vi "Bertta_v09_95.vi"() -> ()   [LabVIEW 2015]
panel:
  out "element":bool
  out "Started:":string
  in  "SHUTDOWN":bool
  in  "MASTER CONTROL":bool
  in  "Tab Control":T1(tab)
  out "Output File":path caption="selected path"
  in  "Browse folder":path=path "" caption="start path"
  in  "Read Seq":bool
  in  "Save Seq":bool
  in  "Configuration file":path=path "C:/Users/shresplab/Desktop/BerttaConfiguration.lvm" caption="Filename"
  in  "OK Button 2":bool
  out "Boolean":bool
  in  "User (initials)":string
  in  "Project name":string
  in  "Description":string
  out "PUMP1":bool
  out "Target amount":dbl
  out "Scale weight":dbl
  out "Amount now":dbl
  out "Flow rate":dbl
  out "Time to target":dbl format="%<%H:%M:%S>t"
  out "Current step":dbl
  out "Target":dbl
  out "Amount now":dbl
  out "Amount now":dbl
  out "Target":dbl
  out "Current step":dbl
  out "Time to target":dbl format="%<%H:%M:%S>t"
  out "Flow rate":dbl
  out "Amount now":dbl
  out "Scale weight":dbl
  out "Target amount":dbl
  out "PUMP2":bool
  out "Sensor OK 6":bool
  out "Sensor OK 5":bool
  out "Sensor OK 4":bool
  out "Sensor OK 3":bool
  in  "OK Button":bool
  in  "Add comment":string
  out "PUMP3":bool
  out "Target amount":dbl
  out "Scale weight":dbl
  out "Amount now":dbl
  out "Flow rate":dbl
  out "Time to target":dbl format="%<%H:%M:%S>t"
  out "Current step":dbl
  out "Target":dbl
  out "Amount now":dbl
  out "Tr":dbl
  out "Tj in":dbl
  out "Tj out":dbl
  out "T set":dbl
  out "Current step":i32
  out "RPM":dbl
  out "Torque 2":dbl
  out "Waveform Chart 5":dynamicdata(graph)
  out "Waveform Chart 6":dynamicdata(graph)
  out "Waveform Chart 7":dynamicdata(graph)
  in  "Tab Control 2":T2(tab)
  out "Waveform Chart 3":dynamicdata(graph)
  out "Waveform Chart 8":dynamicdata(graph)
  out "Waveform Chart 11":dynamicdata(graph)
  out "Waveform Chart 13":dynamicdata(graph)
  out "Waveform Chart 9":dynamicdata(graph)
  out "Table":string[][](table)=[["14.8.2017 18.06.59", "0,000000", "417,670000", "-0,150000", "1,000000", "22,220000", "23,366837", "23,574959", "23,985852", "23,690000", "240,000000", "4,000000", "0,000000", "397,000000", "-397,000000", "1,000000"], ["14.8.2017 18.07.06", "0,000000", "417,640000", "-0,120000", "1,000000", "22,220000", "23,763115", "23,906257", "23,985694", "23,680000", "240,000000", "4,000000", "0,000000", "397,000000", "-397,000000", "1,000000"], ["14.8.2017 18.07.13", "0,000000", "417,640000", "-0,120000", "1,000000", "22,220000", "23,965922", "24,013440", "23,984906", "23,670000", "240,000000", "4,100000", "3,000000", "397,000000", "-397,000000", "1,000000"], ["14.8.2017 18.07.21", "0,000000", "417,640000", "-0,120000", "1,000000", "22,220000", "23,943860", "23,900110", "23,987113", "23,670000", "240,000000", "4,000000", "0,000000", "397,000000", "-397,000000", "1,000000"], ["14.8.2017 18.07.28", "0,000000", "417,640000", "-0,120000", "1,000000", "22,220000", "23,736328", "23,600018", "23,989004", "23,660000", "240,000000", "4,000000", "0,000000", "397,000000", "-397,000000", "1,000000"], ["14.8.2017 18.07.36", "0,000000", "417,640000", "-0,120000", "1,000000", "22,220000", "23,480910", "23,324538", "23,991053", "23,660000", "240,000000", "4,000000", "0,000000", "397,000000", "-397,000000", "1,000000"], ["14.8.2017 18.07.43", "0,000000", "417,640000", "-0,120000", "2,000000", "22,220000", "23,195579", "23,008270", "23,999093", "23,650000", "240,000000", "4,000000", "0,000000", "397,000000", "-397,000000", "1,000000"], ["14.8.2017 18.07.51", "0,000000", "417,650000", "-417,650000", "1,000000", "22,220000", "22,862541", "22,649021", "24,003979", "23,650000", "240,000000", "4,000000", "0,000000", "397,000000", "-397,000000", "2,000000"], ["14.8.2017 18.07.58", "0,000000", "417,640000", "0,010000", "1,000000", "22,220000", "22,541353", "22,354878", "24,005398", "23,650000", "240,000000", "4,000000", "0,000000", "397,000000", "-397,000000", "1,000000"], ["14.8.2017 18.08.06", "0,000000", "417,640000", "0,010000", "1,000000", "22,220000", "22,347931", "22,253738", "24,007605", "23,640000", "240,000000", "4,100000", "0,000000", "397,000000", "-397,000000", "1,000000"], ["14.8.2017 18.08.13", "0,000000", "417,640000", "0,010000", "1,000000", "22,220000", "22,329030", "22,302102", "24,006028", "23,640000", "240,000000", "4,000000", "0,000000", "395,820000", "-395,820000", "1,000000"], ["14.8.2017 18.08.20", "0,000000", "417,640000", "0,010000", "1,000000", "22,220000", "22,466849", "22,511320", "24,002403", "23,630000", "240,000000", "4,000000", "0,000000", "395,830000", "-0,010000", "1,000000"], ["14.8.2017 18.08.28", "0,000000", "417,640000", "0,010000", "1,000000", "22,220000", "22,707062", "22,835101", "24,000984", "23,620000", "240,000000", "4,000000", "0,000000", "395,830000", "-0,010000", "1,000000"], ["14.8.2017 18.08.35", "0,000000", "417,640000", "0,010000", "1,000000", "22,220000", "23,054104", "23,232979", "24,001299", "23,600000", "240,000000", "4,000000", "0,000000", "395,830000", "-0,010000", "1,000000"], ["14.8.2017 18.08.43", "0,000000", "417,640000", "0,010000", "1,000000", "22,220000", "23,412371", "23,522793", "24,002560", "23,590000", "240,000000", "4,000000", "0,000000", "395,820000", "0,000000", "1,000000"], ["14.8.2017 18.08.51", "0,000000", "417,640000", "0,010000", "1,000000", "22,220000", "23,596247", "23,656125", "24,003821", "23,580000", "240,000000", "4,000000", "0,000000", "395,820000", "0,000000", "1,000000"]]
  out "Boolean 4":bool
  out "Boolean 3":bool
  out "Boolean 2":bool
  in  "Reset 6":bool
  in  "Manual/Ramp":bool=TRUE
  in  "Array":dbl[][](array[numeric])=[[20.0, 0.0], [20.0, 0.0], [20.0, 0.0]]
  in  "?":bool
  in  "Time":dbl format="Time to target (min):                %#_g"
  out "Current temp":dbl format="Current temperature (S1):   %#_6g"
  in  "OK Button 3":bool
  in  "T ext / T ext 2":enum32{"Sensor 1", "Sensor 2"}(radio)
  out "Sensor OK":bool
  in  "T fail":dbl=20.0 format="Failsafe temperature:              %#_g"
  in  "Setpoint":dbl=20.0 format="Temperature target:                %#_6g"
  in  "Manual select":T3(radio)
  out "Waveform Chart":dynamicdata(graph)
  out "T external 2":dbl format="Current temperature (S2):    %#_g"
  in  "UPDATE TEMP":bool
  out "Led11 5":bool
  out "RPM":dbl format="%_4f"
  out "Led10 3":bool
  out "Led9 3":bool
  out "Led8 3":bool
  out "Led7 3":bool
  out "Led6 3":bool
  out "Led5 3":bool
  out "Led4 3":bool
  out "Led3 3":bool
  out "Led2 3":bool
  out "Led1 3":bool
  in  "PumpSeq 4":dbl[][](array[numeric])=[[0.0, 0.0, 0.0, 0.0, 0.0, 0.0, 0.0, 0.0, 0.0, 0.0], [0.0, 0.0, 0.0, 0.0, 0.0, 0.0, 0.0, 0.0, 0.0, 0.0], [0.0, 0.0, 0.0, 0.0, 0.0, 0.0, 0.0, 0.0, 0.0, 0.0], [0.0, 0.0, 0.0, 0.0, 0.0, 0.0, 0.0, 0.0, 0.0, 0.0], [0.0, 0.0, 0.0, 0.0, 0.0, 0.0, 0.0, 0.0, 0.0, 0.0], [0.0, 0.0, 0.0, 0.0, 0.0, 0.0, 0.0, 0.0, 0.0, 0.0], [0.0, 0.0, 0.0, 0.0, 0.0, 0.0, 0.0, 0.0, 0.0, 0.0], [0.0, 0.0, 0.0, 0.0, 0.0, 0.0, 0.0, 0.0, 0.0, 0.0], [0.0, 0.0, 0.0, 0.0, 0.0, 0.0, 0.0, 0.0, 0.0, 0.0], [0.0, 0.0, 0.0, 0.0, 0.0, 0.0, 0.0, 0.0, 0.0, 0.0]]
  in  "?":bool
  out "Flow rate (g/min)":dbl
  out "Scale reading":dbl
  out "Step amount now":dbl
  in  "Grams / min":dbl
  out "Waveform Chart 14":dynamicdata(graph)
  in  "?":bool
  out "Total amount now":dbl
  out "Led11 4":bool
  in  "Reset 5":bool
  out "Elapsed / step":i32
  out "Time to target":dbl format="%<%H:%M:%S>t"
  in  "OK Button 4":bool
  out "Led11":bool
  out "RPM":dbl format="%_4f"
  out "Led10":bool
  out "Led9":bool
  out "Led8":bool
  out "Led7":bool
  out "Led6":bool
  out "Led5":bool
  out "Led4":bool
  out "Led3":bool
  out "Led2":bool
  out "Led1":bool
  in  "PumpSeq 2":dbl[][](array[numeric])=[[0.0, 0.0, 0.0, 0.0, 0.0, 0.0, 0.0, 0.0, 0.0, 0.0], [0.0, 0.0, 0.0, 0.0, 0.0, 0.0, 0.0, 0.0, 0.0, 0.0], [0.0, 0.0, 0.0, 0.0, 0.0, 0.0, 0.0, 0.0, 0.0, 0.0], [0.0, 0.0, 0.0, 0.0, 0.0, 0.0, 0.0, 0.0, 0.0, 0.0], [0.0, 0.0, 0.0, 0.0, 0.0, 0.0, 0.0, 0.0, 0.0, 0.0], [0.0, 0.0, 0.0, 0.0, 0.0, 0.0, 0.0, 0.0, 0.0, 0.0], [0.0, 0.0, 0.0, 0.0, 0.0, 0.0, 0.0, 0.0, 0.0, 0.0], [0.0, 0.0, 0.0, 0.0, 0.0, 0.0, 0.0, 0.0, 0.0, 0.0], [0.0, 0.0, 0.0, 0.0, 0.0, 0.0, 0.0, 0.0, 0.0, 0.0], [0.0, 0.0, 0.0, 0.0, 0.0, 0.0, 0.0, 0.0, 0.0, 0.0]]
  in  "?":bool
  out "Flow rate (g/min)":dbl
  out "Scale reading":dbl
  out "Step amount now":dbl
  in  "Grams / min":dbl
  out "Waveform Chart 10":dynamicdata(graph)
  in  "?":bool
  out "Total amount now":dbl
  out "Led11":bool
  in  "Reset 3":bool
  out "Elapsed / step":i32
  out "Time to target":dbl format="%<%H:%M:%S>t"
  in  "OK Button 5":bool
  out "Led11 3":bool
  out "RPM":dbl format="%_4f"
  out "Led10 2":bool
  out "Led9 2":bool
  out "Led8 2":bool
  out "Led7 2":bool
  out "Led6 2":bool
  out "Led5 2":bool
  out "Led4 2":bool
  out "Led3 2":bool
  out "Led2 2":bool
  out "Led1 2":bool
  in  "PumpSeq 3":dbl[][](array[numeric])=[[0.0, 0.0, 0.0, 0.0, 0.0, 0.0, 0.0, 0.0, 0.0, 0.0], [0.0, 0.0, 0.0, 0.0, 0.0, 0.0, 0.0, 0.0, 0.0, 0.0], [0.0, 0.0, 0.0, 0.0, 0.0, 0.0, 0.0, 0.0, 0.0, 0.0], [0.0, 0.0, 0.0, 0.0, 0.0, 0.0, 0.0, 0.0, 0.0, 0.0], [0.0, 0.0, 0.0, 0.0, 0.0, 0.0, 0.0, 0.0, 0.0, 0.0], [0.0, 0.0, 0.0, 0.0, 0.0, 0.0, 0.0, 0.0, 0.0, 0.0], [0.0, 0.0, 0.0, 0.0, 0.0, 0.0, 0.0, 0.0, 0.0, 0.0], [0.0, 0.0, 0.0, 0.0, 0.0, 0.0, 0.0, 0.0, 0.0, 0.0], [0.0, 0.0, 0.0, 0.0, 0.0, 0.0, 0.0, 0.0, 0.0, 0.0], [0.0, 0.0, 0.0, 0.0, 0.0, 0.0, 0.0, 0.0, 0.0, 0.0]]
  in  "?":bool
  out "Flow rate (g/min)":dbl
  out "Scale reading":dbl
  out "Step amount now":dbl
  in  "Grams / min":dbl
  out "Waveform Chart 12":dynamicdata(graph)
  in  "?":bool
  out "Total amount now":dbl
  out "Led11 2":bool
  in  "Reset 4":bool
  out "Elapsed / step":i32
  out "Time to target":dbl format="%<%H:%M:%S>t"
  in  "OK Button 6":bool
  in  "Bypass select 2":enum32{"Remote", "Manual"}(radio)=enum."Manual"
  in  "Port":dbl=13.0
  out "RPM":dbl
  out "Torque":dbl
  in  "Set RPM":dbl(slide) scale=0.0..2000.0
  out "Waveform Chart 4":dynamicdata(graph)
  in  "OK Button 7":bool
  out "PortDev out":dbl[](array[numeric])
  in  "Save PortDev":bool
  out "PortDev in":dbl[](array[numeric])
  in  "dev1":i32
  in  "dev2":i32
  in  "dev3":i32
  in  "dev4":i32
  in  "dev5":i32
  in  "dev6":i32
  in  "dev8":i32
  in  "port1":i32
  in  "port2":i32
  in  "port3":i32
  in  "port4":i32
  in  "port5":i32
  in  "port6":i32
  in  "port7":i32
  in  "port8":i32
  in  "dev7":i32
  in  "Treshold (T/C)":dbl=0.5
  out "DAQ 9217 (PT100)":errorcluster
  out "Config File":dbl[][](array[numeric])
  # "Temperature sensor:"
  # "Manual control:"
  # "PUMP & SCALE 1"
  # "STEP"
  # "TOTAL"
  # "PUMP & SCALE 2"
  # "STEP"
  # "TOTAL"
  # "PUMP & SCALE 3"
  # "STEP"
  # "TOTAL"
  # "Temperature control parameter"
  # "Secondary temperature sensor"
  # "Temp target"
  # "Time target"
  # "Grams    /   min"
  # "End of sequence"
  # "Manual control"
  # "Grams    /   min"
  # "End of sequence"
  # "Manual control"
  # "Grams    /   min"
  # "End of sequence"
  # "Manual control"
  # "dev1 and dev2 always to port1 and 2\nport1 = port2 = Lauda\n\ndev3 and dev4 always to port3 and port4\nport3 = port4 = Heidolph"
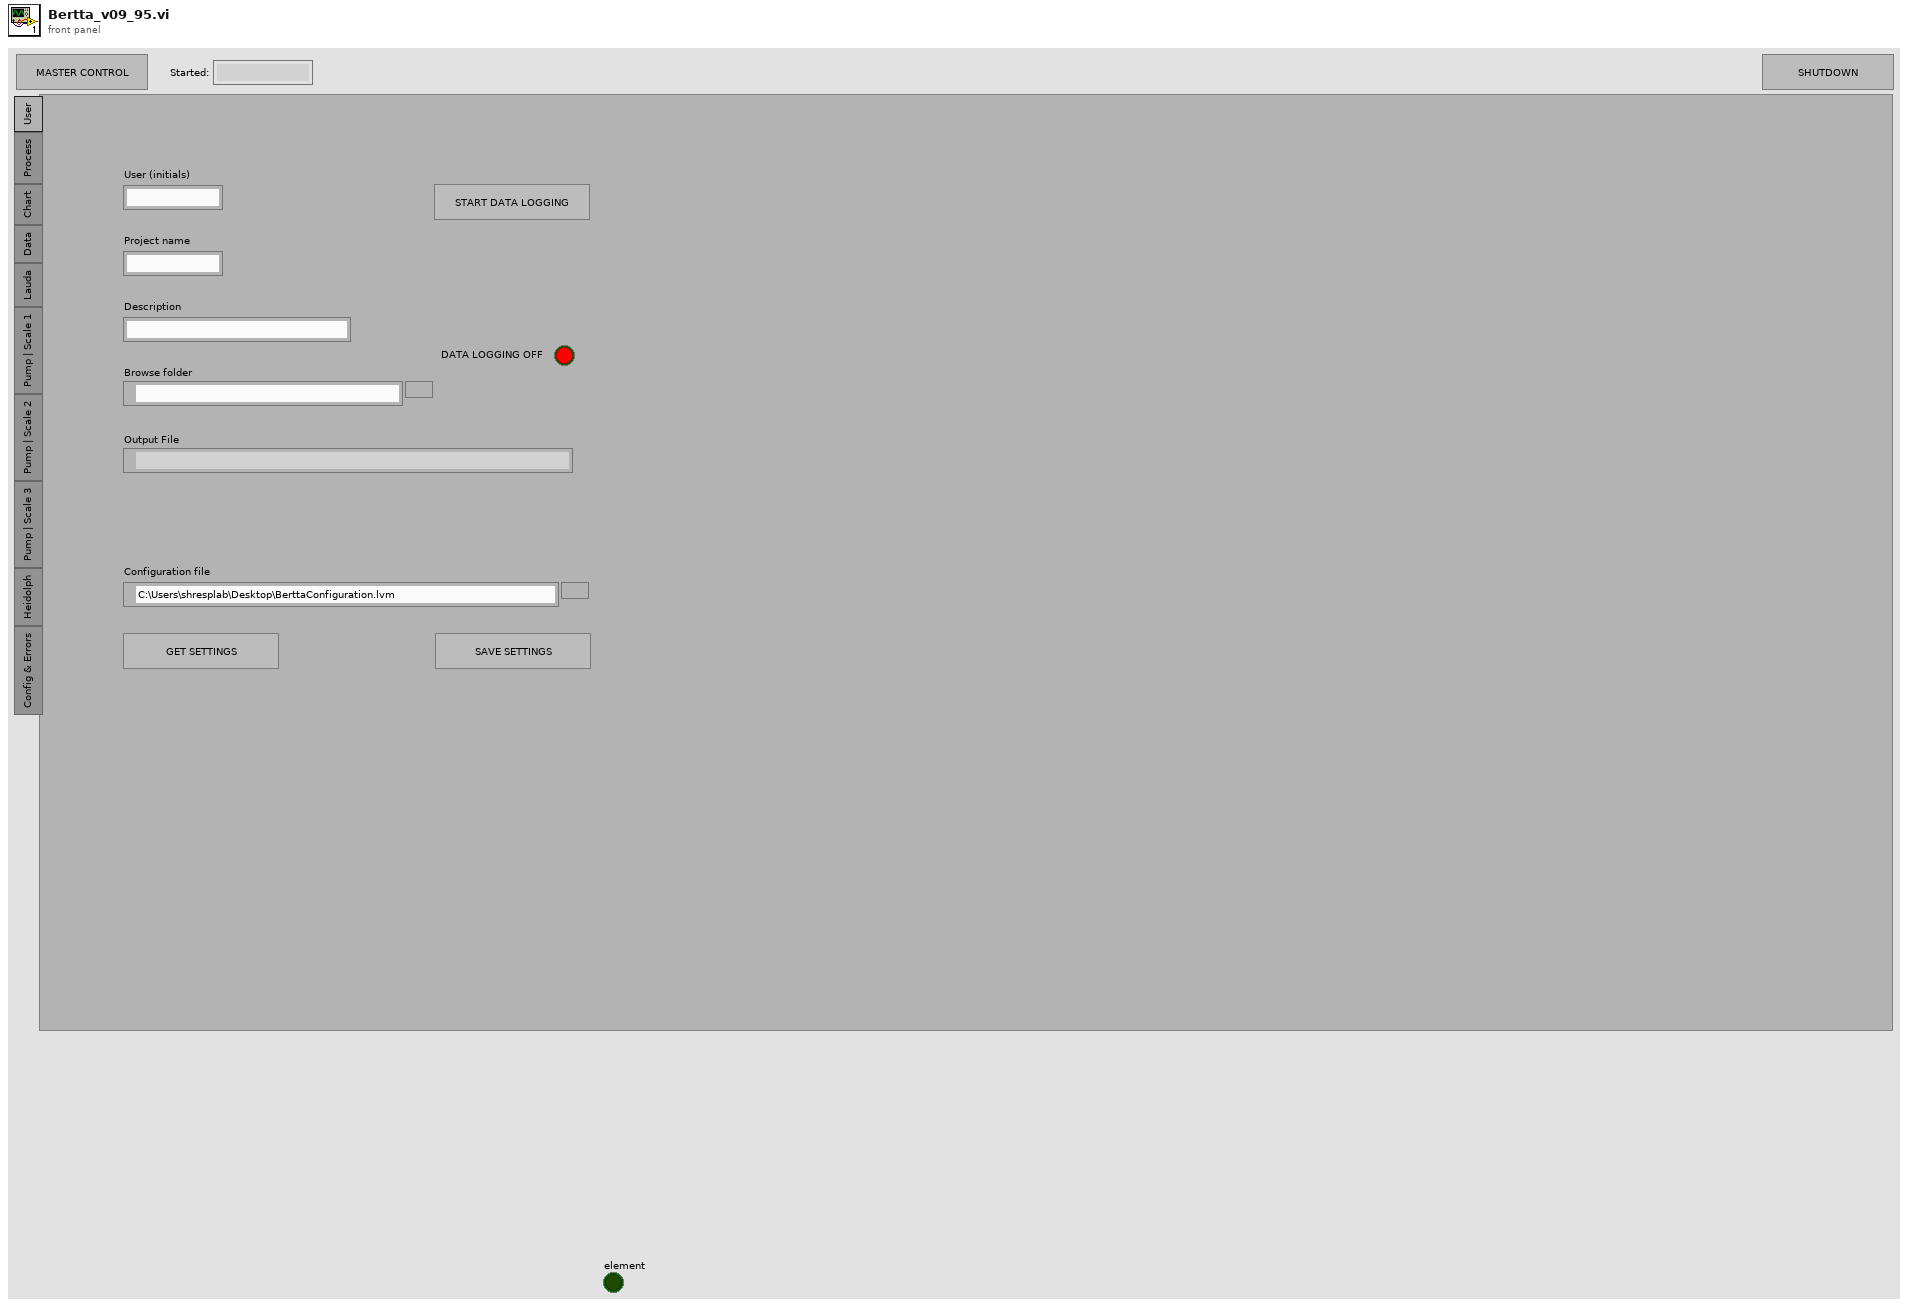
[diagram p1: front panel]
types:
  T1 = enum32{"User", "Process", "Chart", "Data", "Lauda", "Pump | Scale 1", "Pump | Scale 2", "Pump | Scale 3", "Heidolph", "Config & Errors"}
  T2 = enum32{"Temperatures", "Scale / Pump 1", "Scale / Pump 2", "Scale / Pump 3", "RPM / torque"}
  T3 = enum32{"Reactor temperature", "Jacket temperature"}
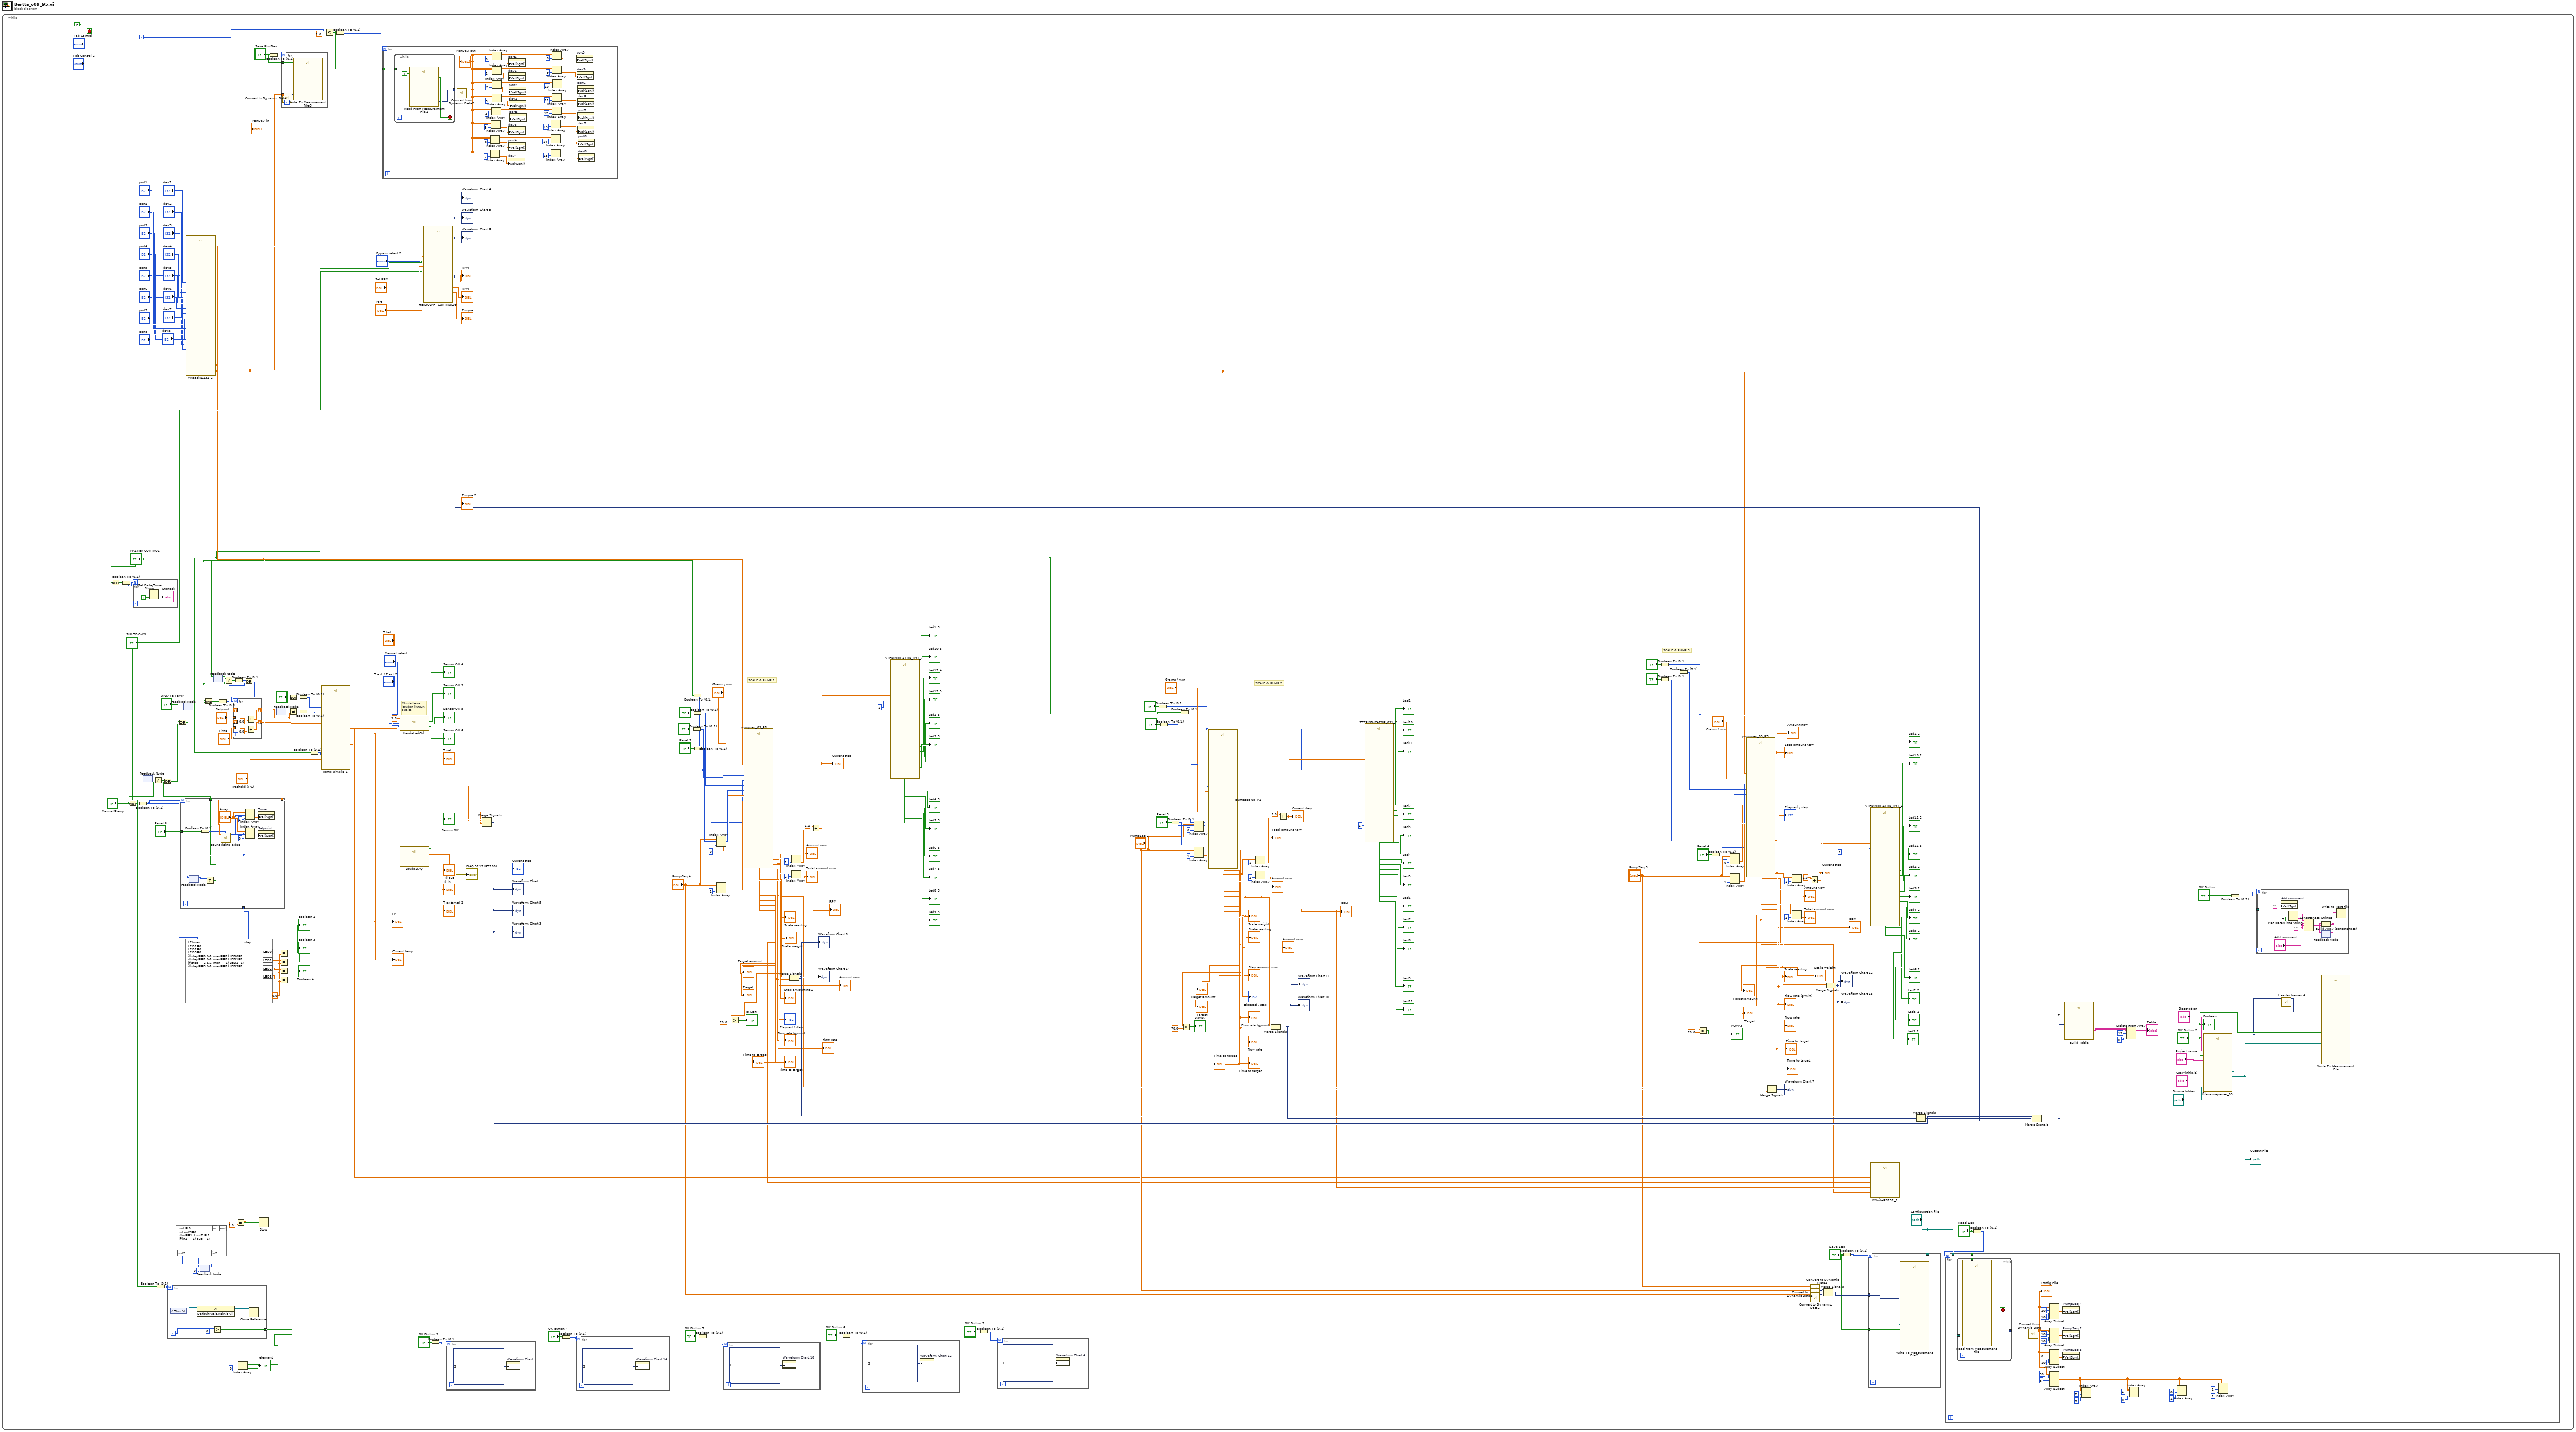
[diagram p0: block diagram]
diagram:
  n1 = while {
    i -> [w28]
    stop <- FALSE stop-if-true
    w14 = 0.0 ("y")
    # "Muutettava\nlaudan kutsun \nosalta"
    # "SCALE & PUMP 1"
    # "SCALE & PUMP 3"
    # "SCALE & PUMP 2"
    n2 = Not(x="MASTER CONTROL") -> (.not. x?=w264:bool)
    n3 = Boolean To (0,1)(Boolean=w264) -> (0, 1=w265:i16)
    n4 = Not(x="Manual/Ramp") -> (.not. x?=w21:bool)
    n5 = for {
      N: w265 -> [_]
      n6 = Get Date/Time String(want seconds? (F)=TRUE) -> (time string=→"Started:":string)  [unwired: 2 in, 1 out]
    }
    n7 = Boolean To (0,1)(Boolean=w21) -> (0, 1=w3:i16)
    n8 = feedback #1() -> (w9:bool)  [unwired: 1 in]
    n9 = feedback-in #1("Manual/Ramp") -> ()
    n10 = Not Equal?(x=w9, y="Manual/Ramp") -> (x != y?=w6:bool)
    n11 = Boolean To (0,1)(Boolean="SHUTDOWN") -> (0, 1=w248:i16)
    n12 = for {
      N: w248 -> [_]
      tunnel: [w381] -> w263 mode=indexing
      i -> [w383]
      n13 = control-ref of="This VI"() -> (w386:refnum<vi>)
      n14 = invoke class="VI" method="Default Vals.Reinit All"(reference=w386) -> (reference out=w384:refnum<vi>, error out=w385:errorcluster)  [unwired: 2 in, 1 out]
      n15 = Greater?(x=w383, y=0) -> (0:w381:bool)
      n16 = Close Reference(reference=w384, error in (no error)=w385) -> ()  [unwired: 1 out]
    }
    n17 = feedback #2() -> (w1:bool)  [unwired: 1 in]
    n18 = call "MReadRS232_2.vi"("port1"="port1", "dev1"="dev1", "port2"="port2", "dev2"="dev2", "port3"="port3", "dev7"="dev7", "dev8"="dev8", "port7"="port7", "port8"="port8", "dev5"="dev5", "port5"="port5", "dev4"="dev4", "dev6"="dev6", "port6"="port6", "port4"="port4", "dev3"="dev3") -> ("output array"=w32:dbl[], "params"=w69:dbl[])  [unwired: 2 in]
    "PortDev in" <- w32
    n19 = feedback #3(0) -> (w246:i32)
    n20 = formula code="out = 0;\nint out2=0;\nif(in==1 ) out2 = 1;\nif(in2==1) out = 1;"("in"=w248, "in2"=w246) -> ("out"=w250:dbl, "out2"=w247:i32)
    n21 = feedback-in #3(w247) -> ()
    n22 = And(x="MASTER CONTROL", y=w1) -> (x .and. y?=w62:bool)
    n23 = feedback #4() -> (w53:bool)  [unwired: 1 in]
    n24 = feedback-in #4("MASTER CONTROL") -> ()
    n25 = Boolean To (0,1)(Boolean=w62) -> (0, 1=w50:i16)
    n26 = Not Equal?(x=w53, y="MASTER CONTROL") -> (x != y?=w52:bool)
    n27 = Boolean To (0,1)(Boolean=w52) -> (0, 1=w49:i16)
    n28 = Equal?(x=w250, y=1.0) -> (x = y?=w249:bool)
    n29 = Index Array(array=w263, index=0) -> (element=→"element":bool)
    n30 = Or(x=w49, y=w50) -> (x .or. y?=w48:i16)
    n31 = for {
      N: w48 -> [_]
      tunnel: "Time" -> [w333]
      shift-right: [w332] -> w63
      shift-left: _ -> [_]
      tunnel: "Setpoint" -> [w330]
      shift-right: [w329] -> w60
      shift-left: _ -> [_]
      n32 = Add(x=w330, y=0.0) -> (x+y=w329:dbl)
      n33 = Add(x=w333, y=0.0) -> (x+y=w332:dbl)
    }
    n34 = Stop(stop? (T)=w249) -> ()
    n35 = Boolean To (0,1)(Boolean="Save PortDev") -> (0, 1=w31:i16)
    n36 = feedback-in #5(w60) -> ()
    n37 = feedback #5() -> (w61:dbl)  [unwired: 1 in]
    n38 = for {
      N: w31 -> [_]
      tunnel: w32 -> [w328]
      tunnel: "Save PortDev" -> [w326]
      n39 = call "Convert to Dynamic Data"("Array"=w328) -> ("Dynamic Data Type"=w327:dynamicdata)  [unwired: 3 in]
      n40 = call "Write To Measurement File3"("Signals"=w327, "Reset"=w326) -> ()  [unwired: 15 in, 3 out]
    }
    n41 = Not(x="?") -> (.not. x?=w56:bool)
    n42 = Not Equal?(x=w61, y=w60) -> (x != y?=w59:bool)
    n43 = Boolean To (0,1)(Boolean=w56) -> (0, 1=w58:i16)
    n44 = Boolean To (0,1)(Boolean=w59) -> (0, 1=w54:i16)
    n45 = Boolean To (0,1)(Boolean="MASTER CONTROL") -> (0, 1=w55:i16)
    n46 = call "ramp_simple_1.vi"("array"=w69, "treshold"="Treshold (T/C)", "time_set"=w63, "T_sp"=w60, "master"=w55, "reset"=w54, "pause"=w58) -> ("T control"=w68:dbl, "Tr"=w67:dbl, "Tin"=w66:dbl, "target_reached"=w19:dbl)  [unwired: 1 out]
    "Tr" <- w67
    "Current temp" <- w67
    n47 = for {
      N: w3 -> [_]
      tunnel: w19 -> [w285]
      tunnel: [w276] -> w7
      tunnel: "Reset 6" -> [w278]
      tunnel: [w277] -> w10
      n48 = feedback #6() -> (w279:i32)  [unwired: 1 in]
      n49 = Boolean To (0,1)(Boolean=w278) -> (0, 1=w280:i16)
      n50 = call "count_rising_edge.vi"("reset"=w280, "target_reached"=w285) -> ("element 2"=w277:i32)  [unwired: 9 in]
      n51 = feedback-in #6(w277) -> ()
      n52 = Not Equal?(x=w279, y=w277) -> (x != y?=w276:bool)
      n53 = Index Array(array="Array", index (row)=w277, index (col)=1 ("disabled index (col)")) -> (element=w281:dbl)
      n54 = Index Array(array="Array", index (row)=w277, index (col)=0 ("disabled index (col)")) -> (element=w282:dbl)
      n55 = property on="Time" class="DigNum (strict)"("Val(Sgnl)"=w281) -> ()  [unwired: 2 in, 2 out]
      n56 = property on="Setpoint" class="DigNum (strict)"("Val(Sgnl)"=w282) -> ()  [unwired: 2 in, 2 out]
    }
    n57 = Or(x=w6, y=w7) -> (x .or. y?=w5:bool)
    n58 = Or(x="UPDATE TEMP", y=w5) -> (x .or. y?=w2:bool)
    n59 = feedback-in #2(w2) -> ()
    n60 = formula code="LED0=0;\nLED1=0;\nLED2=0;\nLED3=0;\nif(step==0 && man==1) LED0=1;\nif(step==1 && man==1) LED1=1;\nif(step==2 && man==1) LED2=1;\nif(step==3 && man==1) LED3=1;"("step"=w10, "man"=w3) -> ("LED0"=w18:dbl, "LED1"=w17:dbl, "LED2"=w16:dbl, "LED3"=w15:dbl)
    n61 = Not Equal?(x=w18, y=w14) -> (x != y?=→"Boolean 2":bool)
    n62 = Not Equal?(x=w17, y=w14) -> (x != y?=→"Boolean 3":bool)
    n63 = Not Equal?(x=w16, y=w14) -> (x != y?=→"Boolean 4":bool)
    n64 = Not Equal?(x=w15, y=w14) -> ()  [unwired: 1 out]
    n65 = Less?(x=w28, y=1.0) -> (x < y?=w26:bool)
    n66 = Boolean To (0,1)(Boolean=w26) -> (0, 1=w27:i16)
    n67 = for {
      N: w27 -> [_]
      tunnel: w26 -> [w321]
      n68 = while {
        tunnel: [w324] -> w320
        tunnel: w321 -> [w322]
        stop <- w325 stop-if-true
        n69 = call "Read From Measurement File2"("Enable"=TRUE, "Reset"=w322) -> ("Signals"=w324:dynamicdata, "EOF?"=w325:bool)  [unwired: 4 in, 4 out]
      }
      n70 = call "Convert from Dynamic Data2"("Dynamic Data Type"=w320) -> ("Array"=w303:dbl[])  [unwired: 3 in]
      "PortDev out" <- w303
      n71 = Index Array(array=w303, index=6) -> (element=w296:dbl)
      n72 = Index Array(array=w303, index=7) -> (element=w295:dbl)
      n73 = Index Array(array=w303, index=5) -> (element=w297:dbl)
      n74 = Index Array(array=w303, index=4) -> (element=w298:dbl)
      n75 = Index Array(array=w303, index=0) -> (element=w302:dbl)
      n76 = Index Array(array=w303, index=1) -> (element=w301:dbl)
      n77 = Index Array(array=w303, index=3) -> (element=w299:dbl)
      n78 = Index Array(array=w303, index=2) -> (element=w300:dbl)
      n79 = property on="dev4" class="DigNum (strict)"("Val(Sgnl)"=w295) -> ()  [unwired: 2 in, 2 out]
      n80 = property on="dev3" class="DigNum (strict)"("Val(Sgnl)"=w297) -> ()  [unwired: 2 in, 2 out]
      n81 = property on="port4" class="DigNum (strict)"("Val(Sgnl)"=w296) -> ()  [unwired: 2 in, 2 out]
      n82 = property on="port1" class="DigNum (strict)"("Val(Sgnl)"=w302) -> ()  [unwired: 2 in, 2 out]
      n83 = property on="dev1" class="DigNum (strict)"("Val(Sgnl)"=w301) -> ()  [unwired: 2 in, 2 out]
      n84 = property on="port2" class="DigNum (strict)"("Val(Sgnl)"=w300) -> ()  [unwired: 2 in, 2 out]
      n85 = property on="dev2" class="DigNum (strict)"("Val(Sgnl)"=w299) -> ()  [unwired: 2 in, 2 out]
      n86 = property on="port3" class="DigNum (strict)"("Val(Sgnl)"=w298) -> ()  [unwired: 2 in, 2 out]
      n87 = Index Array(array=w303, index=14) -> (element=w288:dbl)
      n88 = Index Array(array=w303, index=15) -> (element=w287:dbl)
      n89 = Index Array(array=w303, index=13) -> (element=w289:dbl)
      n90 = Index Array(array=w303, index=12) -> (element=w290:dbl)
      n91 = Index Array(array=w303, index=8) -> (element=w294:dbl)
      n92 = Index Array(array=w303, index=9) -> (element=w293:dbl)
      n93 = Index Array(array=w303, index=11) -> (element=w291:dbl)
      n94 = Index Array(array=w303, index=10) -> (element=w292:dbl)
      n95 = property on="port5" class="DigNum (strict)"("Val(Sgnl)"=w294) -> ()  [unwired: 2 in, 2 out]
      n96 = property on="dev5" class="DigNum (strict)"("Val(Sgnl)"=w293) -> ()  [unwired: 2 in, 2 out]
      n97 = property on="port6" class="DigNum (strict)"("Val(Sgnl)"=w292) -> ()  [unwired: 2 in, 2 out]
      n98 = property on="dev6" class="DigNum (strict)"("Val(Sgnl)"=w291) -> ()  [unwired: 2 in, 2 out]
      n99 = property on="port7" class="DigNum (strict)"("Val(Sgnl)"=w290) -> ()  [unwired: 2 in, 2 out]
      n100 = property on="dev7" class="DigNum (strict)"("Val(Sgnl)"=w289) -> ()  [unwired: 2 in, 2 out]
      n101 = property on="port8" class="DigNum (strict)"("Val(Sgnl)"=w288) -> ()  [unwired: 2 in, 2 out]
      n102 = property on="dev8" class="DigNum (strict)"("Val(Sgnl)"=w287) -> ()  [unwired: 2 in, 2 out]
    }
    n103 = call "LaudaLedCtrl.vi"("Manual select"="Manual select", "T ext / T ext in"="T ext / T ext 2", "Lauda port"=9.0) -> ("Sensor OK 5"=→"Sensor OK 5":bool, "Sensor OK 3"=→"Sensor OK 3":bool, "Sensor OK 4"=→"Sensor OK 4":bool, "Sensor OK 6"=→"Sensor OK 6":bool)  [unwired: 5 in]
    n104 = call "LaudaDAQ.vi"() -> ("error out"=→"DAQ 9217 (PT100)":errorcluster, 1:"Tj out"=→"Tj out":dbl, "data"=w137:dynamicdata, "Sensor OK"=→"Sensor OK":bool, 4:"Tj out"=→"Tj in":dbl, "T external 2"=→"T external 2":dbl)  [unwired: 6 in]
    n105 = call "HEIDOLPH_CONTROL09.vi"("master"="MASTER CONTROL", "Array"=w69, "shutdown"="SHUTDOWN", "Bypass select"="Bypass select 2", "Set RPM"="Set RPM", "Device port"="Port") -> ("Dynamic Data"=w138:dynamicdata, "RPM"=→"RPM":dbl, "RPM 2"=→"RPM":dbl, "Torque"=→"Torque":dbl, "Torque 2"=→"Torque 2":dbl)  [unwired: 1 in]
    "Waveform Chart 4" <- w138
    "Waveform Chart 6" <- w138
    "Waveform Chart 9" <- w138
    n106 = Boolean To (0,1)(Boolean="OK Button 3") -> (0, 1=w80:i16)
    n107 = for {
      N: w80 -> [_]
      n108 = property on="Waveform Chart" class="WFChart (strict)"("History Data"=dynamicdata[] []) -> ()  [unwired: 2 in, 2 out]
    }
    n109 = Merge Signals(w68, w67, w66, w137) -> (w139:dynamicdata)
    "Waveform Chart 3" <- w139
    "Waveform Chart" <- w139
    "Waveform Chart 5" <- w139
    n110 = Boolean To (0,1)(Boolean="OK Button 4") -> (0, 1=w78:i16)
    n111 = for {
      N: w78 -> [_]
      n112 = property on="Waveform Chart 14" class="WFChart (strict)"("History Data"=dynamicdata[] []) -> ()  [unwired: 2 in, 2 out]
    }
    n113 = Boolean To (0,1)(Boolean="?") -> (0, 1=w147:i16)
    n114 = Boolean To (0,1)(Boolean="?") -> (0, 1=w151:i16)
    n115 = Boolean To (0,1)(Boolean="MASTER CONTROL") -> (0, 1=w143:i16)
    n116 = Boolean To (0,1)(Boolean="Reset 5") -> (0, 1=w150:i16)
    n117 = Boolean To (0,1)(Boolean="OK Button 5") -> (0, 1=w76:i16)
    n118 = Index Array(array="PumpSeq 4", index (col)=0) -> (element=w155:dbl[])  [unwired: 1 in]
    n119 = Index Array(array="PumpSeq 4", index (col)=1) -> (element=w176:dbl[])  [unwired: 1 in]
    n120 = for {
      N: w76 -> [_]
      n121 = property on="Waveform Chart 10" class="WFChart (strict)"("History Data"=dynamicdata[] []) -> ()  [unwired: 2 in, 2 out]
    }
    n122 = call "pumpsec_09_P1.vi"("reset"=w150, "master"=w143, "manual"=w147, "pause"=w151, "Array"=w69, "Target"=w155, "fr_manual"="Grams / min", "Time"=w176) -> ("pumpCtrl"=w121:dbl, "totaltarget"=→"Target":dbl, "target_step"=→"Target amount":dbl, "REGLO D"=w87:dbl, "time_to_target"=→"Time to target" →"Time to target":dbl, "step_fr"=w98:dbl, "amount_step"=→"Amount now" →"Step amount now":dbl, "Scale"=w133:dbl, "elapsed_step"=→"Elapsed / step":dbl, "params"=w173:dbl[])  [unwired: 8 in, 2 out]
    "Flow rate" <- w98
    "Scale weight" <- w133
    "Scale reading" <- w133
    "Flow rate (g/min)" <- w98
    "RPM" <- w87
    n123 = Greater?(x=w121, y=70.0) -> (0:→"PUMP1":bool)
    n124 = Merge Signals(w133, w98) -> (w142:dynamicdata)
    "Waveform Chart 8" <- w142
    "Waveform Chart 14" <- w142
    n125 = Index Array(array=w173, index=1) -> (element=w170:dbl)
    n126 = Index Array(array=w173, index=2) -> (element=→"Amount now" →"Total amount now":dbl)
    n127 = Add(x=1.0, y=w170) -> (x+y=w99:dbl)
    "Current step" <- w99
    n128 = Boolean To (0,1)(Boolean="OK Button 6") -> (0, 1=w74:i16)
    n129 = for {
      N: w74 -> [_]
      n130 = property on="Waveform Chart 12" class="WFChart (strict)"("History Data"=dynamicdata[] []) -> ()  [unwired: 2 in, 2 out]
    }
    n131 = call "STEPINDICATOR_091_2.vi"("current step"=w99, "enable"=i16 1, "manual"=w147) -> ("Led 8"=→"Led8 3":bool, "Led 10"=→"Led10 3":bool, "Led 11"=→"Led11 4":bool, "Led 7"=→"Led7 3":bool, "Led 1"=→"Led1 3":bool, "Led 6"=→"Led6 3":bool, "Led 2"=→"Led2 3":bool, "Led 12"=→"Led11 5":bool, "Led 5"=→"Led5 3":bool, "Led 4"=→"Led4 3":bool, "Led 3"=→"Led3 3":bool, "Led 9"=→"Led9 3":bool)  [unwired: 1 in]
    n132 = Boolean To (0,1)(Boolean="OK Button 7") -> (0, 1=w72:i16)
    n133 = for {
      N: w72 -> [_]
      n134 = property on="Waveform Chart 4" class="WFChart (strict)"("History Data"=dynamicdata[] []) -> ()  [unwired: 2 in, 2 out]
    }
    n135 = Boolean To (0,1)(Boolean="?") -> (0, 1=w210:i16)
    n136 = Boolean To (0,1)(Boolean="?") -> (0, 1=w237:i16)
    n137 = Boolean To (0,1)(Boolean="Reset 3") -> (0, 1=w235:i16)
    n138 = Boolean To (0,1)(Boolean="MASTER CONTROL") -> (0, 1=w229:i16)
    n139 = Index Array(array="PumpSeq 2", index (col)=0 ("disabled index (col)")) -> (element=w240:dbl[])  [unwired: 1 in]
    n140 = Index Array(array="PumpSeq 2", index (col)=1 ("disabled index (col)")) -> (element=w239:dbl[])  [unwired: 1 in]
    n141 = call "pumpsec_09_P2.vi"("reset"=w235, "master"=w229, "manual"=w210, "pause"=w237, "Array"=w69, "Target"=w240, "fr_manual"="Grams / min", "Time"=w239) -> ("pumpCtrl"=w117:dbl, "totaltarget"=→"Target":dbl, "target_step"=→"Target amount":dbl, "REGLO D"=w86:dbl, "time_to_target"=→"Time to target" →"Time to target":dbl, "step_fr"=w136:dbl, "amount_step"=→"Amount now" →"Step amount now":dbl, "Scale"=w132:dbl, "elapsed_step"=→"Elapsed / step":dbl, "params"=w230:dbl[])  [unwired: 8 in, 2 out]
    "Scale weight" <- w132
    "Flow rate" <- w136
    "Scale reading" <- w132
    "Flow rate (g/min)" <- w136
    "RPM" <- w86
    n142 = Greater?(x=w117, y=70.0) -> (0:→"PUMP2":bool)
    n143 = Index Array(array=w230, index=1) -> (element=w233:dbl)
    n144 = Index Array(array=w230, index=2) -> (element=→"Amount now" →"Total amount now":dbl)
    n145 = Merge Signals(w132, w136) -> (w144:dynamicdata)
    "Waveform Chart 11" <- w144
    "Waveform Chart 10" <- w144
    n146 = Add(x=1.0, y=w233) -> (x+y=w227:dbl)
    "Current step" <- w227
    n147 = call "STEPINDICATOR_091_2.vi"("current step"=w227, "enable"=i16 1, "manual"=w210) -> ("Led 8"=→"Led8":bool, "Led 10"=→"Led10":bool, "Led 11"=→"Led11":bool, "Led 7"=→"Led7":bool, "Led 1"=→"Led1":bool, "Led 6"=→"Led6":bool, "Led 2"=→"Led2":bool, "Led 12"=→"Led11":bool, "Led 5"=→"Led5":bool, "Led 4"=→"Led4":bool, "Led 3"=→"Led3":bool, "Led 9"=→"Led9":bool)  [unwired: 1 in]
    n148 = Boolean To (0,1)(Boolean="?") -> (0, 1=w204:i16)
    n149 = Boolean To (0,1)(Boolean="?") -> (0, 1=w203:i16)
    n150 = Boolean To (0,1)(Boolean="MASTER CONTROL") -> (0, 1=w205:i16)
    n151 = Boolean To (0,1)(Boolean="Reset 4") -> (0, 1=w185:i16)
    n152 = Index Array(array="PumpSeq 3", index (col)=0 ("disabled index (col)")) -> (element=w188:dbl[])  [unwired: 1 in]
    n153 = Index Array(array="PumpSeq 3", index (col)=1 ("disabled index (col)")) -> (element=w187:dbl[])  [unwired: 1 in]
    n154 = call "pumpsec_09_P3.vi"("reset"=w185, "master"=w205, "manual"=w204, "pause"=w203, "Array"=w69, "Target"=w188, "fr_manual"="Grams / min", "Time"=w187) -> ("pumpCtrl"=w114:dbl, "totaltarget"=→"Target":dbl, "target_step"=→"Target amount":dbl, "REGLO D"=w85:dbl, "time_to_target"=→"Time to target" →"Time to target":dbl, "step_fr"=w135:dbl, "amount_step"=→"Amount now" →"Step amount now":dbl, "Scale"=w131:dbl, "elapsed_step"=→"Elapsed / step":dbl, "params"=w178:dbl[])  [unwired: 8 in, 2 out]
    "Scale weight" <- w131
    "Flow rate" <- w135
    "Scale reading" <- w131
    "Flow rate (g/min)" <- w135
    "RPM" <- w85
    n155 = Greater?(x=w114, y=70.0) -> (0:→"PUMP3":bool)
    n156 = Merge Signals(w133, w132, w131) -> (→"Waveform Chart 7":dynamicdata)
    n157 = Index Array(array=w178, index=1) -> (element=w179:dbl)
    n158 = Index Array(array=w178, index=2) -> (element=→"Amount now" →"Total amount now":dbl)
    n159 = Add(x=1.0, y=w179) -> (x+y=w177:dbl)
    "Current step" <- w177
    n160 = call "Convert to Dynamic Data4"("2D Array"="PumpSeq 3") -> ("Dynamic Data Type"=w90:dynamicdata)  [unwired: 3 in]
    n161 = call "Convert to Dynamic Data3"("2D Array"="PumpSeq 2") -> ("Dynamic Data Type"=w92:dynamicdata)  [unwired: 3 in]
    n162 = call "Convert to Dynamic Data2"("2D Array"="PumpSeq 4") -> ("Dynamic Data Type"=w95:dynamicdata)  [unwired: 3 in]
    n163 = Merge Signals(w90, w92, w95) -> (w94:dynamicdata)
    n164 = Merge Signals(w131, w135) -> (w141:dynamicdata)
    "Waveform Chart 13" <- w141
    "Waveform Chart 12" <- w141
    n165 = Boolean To (0,1)(Boolean="Save Seq") -> (0, 1=w89:i16)
    n166 = for {
      N: w89 -> [_]
      tunnel: w94 -> [w379]
      tunnel: "Configuration file" -> [w380]
      tunnel: "Save Seq" -> [w378]
      n167 = call "Write To Measurement File2"("Signals"=w379, "Reset"=w378, "Filename"=w380) -> ()  [unwired: 14 in, 3 out]
    }
    n168 = call "STEPINDICATOR_091_4.vi"("current step"=w177, "enable"=i16 1, "manual"=w204) -> ("Led 8"=→"Led8 2":bool, "Led 10"=→"Led10 2":bool, "Led 11"=→"Led11 2":bool, "Led 7"=→"Led7 2":bool, "Led 1"=→"Led1 2":bool, "Led 6"=→"Led6 2":bool, "Led 2"=→"Led2 2":bool, "Led 12"=→"Led11 3":bool, "Led 5"=→"Led5 2":bool, "Led 4"=→"Led4 2":bool, "Led 3"=→"Led3 2":bool, "Led 9"=→"Led9 2":bool)  [unwired: 1 in]
    n169 = call "MWriteRS232_1.vi"("P3"=w85, "P2"=w86, "P1"=w87, "LAUDA"=w68) -> ()  [unwired: 8 in]
    n170 = Merge Signals(w142, w144, w141) -> (w140:dynamicdata)
    n171 = Boolean To (0,1)(Boolean="Read Seq") -> (0, 1=w88:i16)
    n172 = for {
      N: w88 -> [_]
      tunnel: "Configuration file" -> [w351]
      tunnel: "Read Seq" -> [w350]
      n173 = while {
        tunnel: [w377] -> w373
        tunnel: w351 -> [w376]
        tunnel: w350 -> [w374]
        stop <- w375 stop-if-true
        n174 = call "Read From Measurement File"("Filename"=w376, "Reset"=w374) -> ("Signals"=w377:dynamicdata, "EOF?"=w375:bool)  [unwired: 4 in, 4 out]
      }
      n175 = call "Convert from Dynamic Data"("Dynamic Data Type"=w373) -> ("Array"=w363:dbl[][])  [unwired: 3 in]
      "Config File" <- w363
      n176 = Array Subset(array=w363, index (row)=20 ("index"), length (row)=10 ("length")) -> (w370:dbl[][])  [unwired: 2 in]
      n177 = Array Subset(array=w363, index (row)=10 ("index"), length (row)=10 ("length")) -> (w365:dbl[][])  [unwired: 2 in]
      n178 = Array Subset(array=w363, index (row)=0 ("index"), length (row)=10 ("length")) -> (w364:dbl[][])  [unwired: 2 in]
      n179 = Array Subset(array=w363, index (row)=30 ("index"), length (row)=8 ("length")) -> (w352:dbl[][])  [unwired: 2 in]
      n180 = property on="PumpSeq 4" class="Arr (strict)"("Val(Sgnl)"=w370) -> ()  [unwired: 2 in, 2 out]
      n181 = property on="PumpSeq 2" class="Arr (strict)"("Val(Sgnl)"=w365) -> ()  [unwired: 2 in, 2 out]
      n182 = property on="PumpSeq 3" class="Arr (strict)"("Val(Sgnl)"=w364) -> ()  [unwired: 2 in, 2 out]
      n183 = Index Array(array=w352, index (row)=2, index (col)=0 ("disabled index (col)")) -> ()  [unwired: 1 out]
      n184 = Index Array(array=w352, index (row)=4, index (col)=0 ("disabled index (col)")) -> ()  [unwired: 1 out]
      n185 = Index Array(array=w352, index (row)=0, index (col)=1 ("disabled index (col)")) -> ()  [unwired: 1 out]
      n186 = Index Array(array=w352, index (row)=1, index (col)=1 ("disabled index (col)")) -> ()  [unwired: 1 out]
    }
    n187 = Merge Signals(w139, w140, w138) -> (w24:dynamicdata)
    n188 = call "Build Table"("Include time data"=TRUE, "Signals"=w24) -> ("Table"=w258:string[][])  [unwired: 3 in, 6 out]
    n189 = Delete From Array(array=w258, length=13, index (col)=0 ("index (row)")) -> (array with subset deleted=→"Table":string[][])  [unwired: 1 in, 1 out]
    n190 = call "filenameparser_09.vi"("Description"="Description", "start path"="Browse folder", "Project name"="Project name", "User (initials)"="User (initials)", "OK Button in"="OK Button 2") -> ("appended path 2"=w70:path, "appended path"=w254:path)  [unwired: 4 in, 1 out]
    "Output File" <- w70
    n191 = Boolean To (0,1)(Boolean="OK Button") -> (0, 1=w253:i16)
    n192 = for {
      N: w253 -> [_]
      tunnel: w254 -> [w342]
      w346 = " " ("string")
      n193 = property on="Add comment" class="Str"("Val(Sgnl)"="" ("Value (Signaling)")) -> ()  [unwired: 2 in, 2 out]
      n194 = Get Date/Time String(want seconds? (F)=TRUE) -> (date string=w349:string, time string=w347:string)  [unwired: 2 in]
      n195 = Concatenate Strings(w349, w346, w347, w346, "Add comment") -> (w345:string)
      n196 = feedback #7() -> (w344:string[])  [unwired: 1 in]
      n197 = Build Array (concatenate)(w344, w345) -> (w343:string[])
      n198 = feedback-in #7(w343) -> ()
      n199 = Write to Text File(file (use dialog)=w342, text=w343) -> ()  [unwired: 2 in, 3 out]
    }
    n200 = call "Header Names 4.vi"("Dynamic Data"=w24) -> ("Signals Out"=w25:dynamicdata)  [unwired: 10 in]
    n201 = call "Write To Measurement File"("Signals"=w25, "Enable"="OK Button 2", "Filename"=w70) -> ()  [unwired: 14 in, 3 out]
    "Boolean" <- "OK Button 2"
  }
